vi "Initialize.vi"(0 "NSIS_Installer in":refnum<class "Compound_Installer.lvclass">) -> (4 "NSIS_Installer out":refnum<class "Compound_Installer.lvclass">)   [LabVIEW 2017, in "CL_G3_VIComponentBuilder.lvlib" / "Compound_Installer.lvclass"]
doc: "Responsible for determining the Unique Name, Product Name, and Export's Build Specification file."
uses:
  Compound_Installer.lvclass
  Exports/Export.lvclass
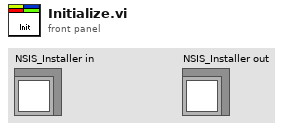
[diagram p1: front panel]
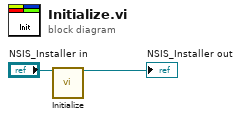
[diagram p0: block diagram]
diagram:
  n1 = call-parent "Initialize.vi"("Export in"="NSIS_Installer in") -> ("Export out"=→"NSIS_Installer out":refnum<class "Compound_Installer.lvclass">)  [unwired: 14 in]
